vi "timeGlobal.vi"() -> ()   [LabVIEW 2016]
panel:
  in  "time_elapsed":dbl
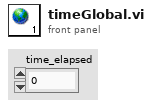
[diagram p1: front panel]
diagram:
